vi "例4.18 同时停止两个While循环.vi"() -> ()   [LabVIEW 2017]
panel:
  out "循环2里的值":dbl
  out "循环1里的值":dbl
  in  "停止":bool
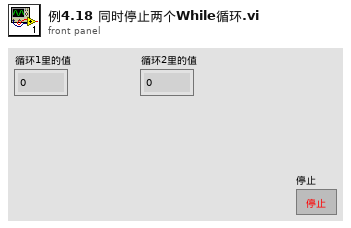
[diagram p1: front panel]
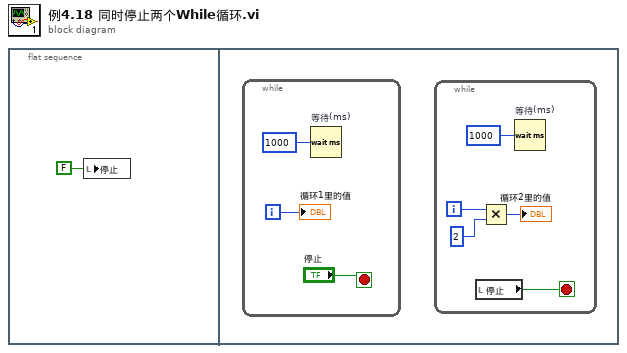
[diagram p0: block diagram]
diagram:
  n1 = flat-sequence {
    frame #0 {
      n2 = local write "停止"(FALSE ("停止")) -> ()
    }
    frame #1 {
      n3 = while {
        i -> [w2]
        stop <- "停止" stop-if-true
        n4 = Wait (ms) "等待(ms)"(milliseconds to wait=u32 1000 ("等待时间（毫秒）")) -> ()  [unwired: 1 out]
        "循环1里的值" <- w2
      }
      n5 = while {
        i -> [w6]
        stop <- w9 stop-if-true
        n6 = local read "停止"() -> (w9:bool)
        n7 = Multiply(x=w6, y=2) -> (x*y=→"循环2里的值":i32)
        n8 = Wait (ms) "等待(ms)"(milliseconds to wait=u32 1000 ("等待时间（毫秒）")) -> ()  [unwired: 1 out]
      }
    }
  }
